vi "DataReceived_CB.vi"(4 "User Parameter":variant, 5 "Event Data":cluster{"p0":refnum<k24>, "p1":refnum<k24>}, 6 "Control Ref":refnum<k24>, 7 "Event Common Data":T1) -> ()   [LabVIEW 2012]
uses:
  C:/Program Files/LeddarTech/xtec/LeddarNET2.dll
  Globals.vi
panel:
  # "These inputs are mandatory and are automatically created\nby LabVIEW when we ask him to \"Create Callback VI\" from the\n\"Register Event Callback\" block."
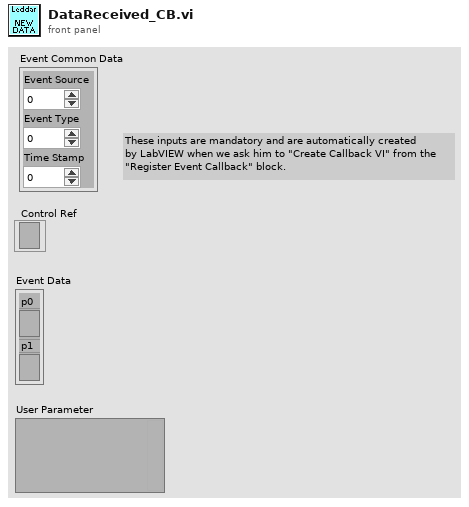
[diagram p1: front panel]
types:
  T1 = cluster{"Event Source":i32, "Event Type":u32, "Time Stamp":u32}
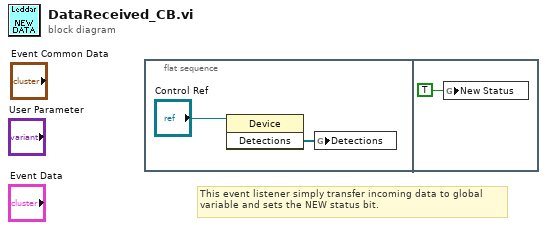
[diagram p0: block diagram]
diagram:
  # "This event listener simply transfer incoming data to global\nvariable and sets the NEW status bit."
  n1 = flat-sequence {
    frame #0 {
      n2 = invoke class="Device" method="Detections"(reference="Control Ref") -> ("Detections"=w2:refnum<k24>[])  [unwired: 2 in, 2 out]
      n3 = global write "Globals.vi" "Detections"(w2) -> ()
    }
    frame #1 {
      n4 = global write "Globals.vi" "New Status"(TRUE) -> ()
    }
  }
